vi "RobotOpen.vi"(8 "error in (no error)":errorcluster, 9 "RobotType":T1, 11 "Robot Communication port name":refnum<visa-resource-name>="ASRL2::INSTR") -> (0 "error out":errorcluster, 3 "Robot Communication port name out":refnum<visa-resource-name>)   [LabVIEW 2014]
doc: "Open UART serial port and initilize iRobot."
uses:
  RobotType.ctl
  <vilib>/myRIO/Instrument Drivers/Onboard IO/UART/typedef/VISA Configuration.ctl
  <vilib>/Instr/_visa.llb/VISA Flush IO Buffer Mask.ctl
  iRobot/Actuator/LED.ctl
  iRobot/Advanced/Command/Baud.ctl
  <vilib>/Instr/_visa.llb/VISA Configure Serial Port (Instr).vi
  <vilib>/myRIO/Instrument Drivers/Onboard IO/UART/UART.lvlib
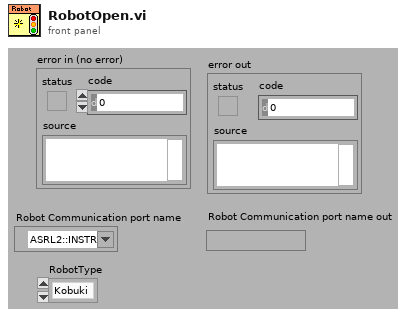
[diagram p1: front panel]
types:
  T1 = typedef "RobotType.ctl" = enum16{"Kobuki", "iRobot"}
  T2 = typedef "Baud.ctl" = enum8{"300", "600", "1200", "2400", "4800", "9600", "14400", "19200", "28800", "38400", "57600", "115200"}
  T3 = typedef "VISA Flush IO Buffer Mask.ctl" = u16
  T4 = typedef "UART.lvlib/VISA Configuration.ctl" = cluster{"baud rate (9600)":u32, "data bits (8)":u16, "parity (0:none)":enum16{"None", "Odd", "Even", "Mark", "Space"}, "stop bits (10: 1 bit)":u16, "flow control (0:none)":u16, "termination char\n(0xA = '\\n' = LF) ":u8, "Enable Termination\nChar (T)":bool, "timeout (10sec)":u32}
  T5 = typedef "LED.ctl" = u8
  T6 = typedef "iRobot UART Port Type.ctl" = refnum<visa-resource-name>
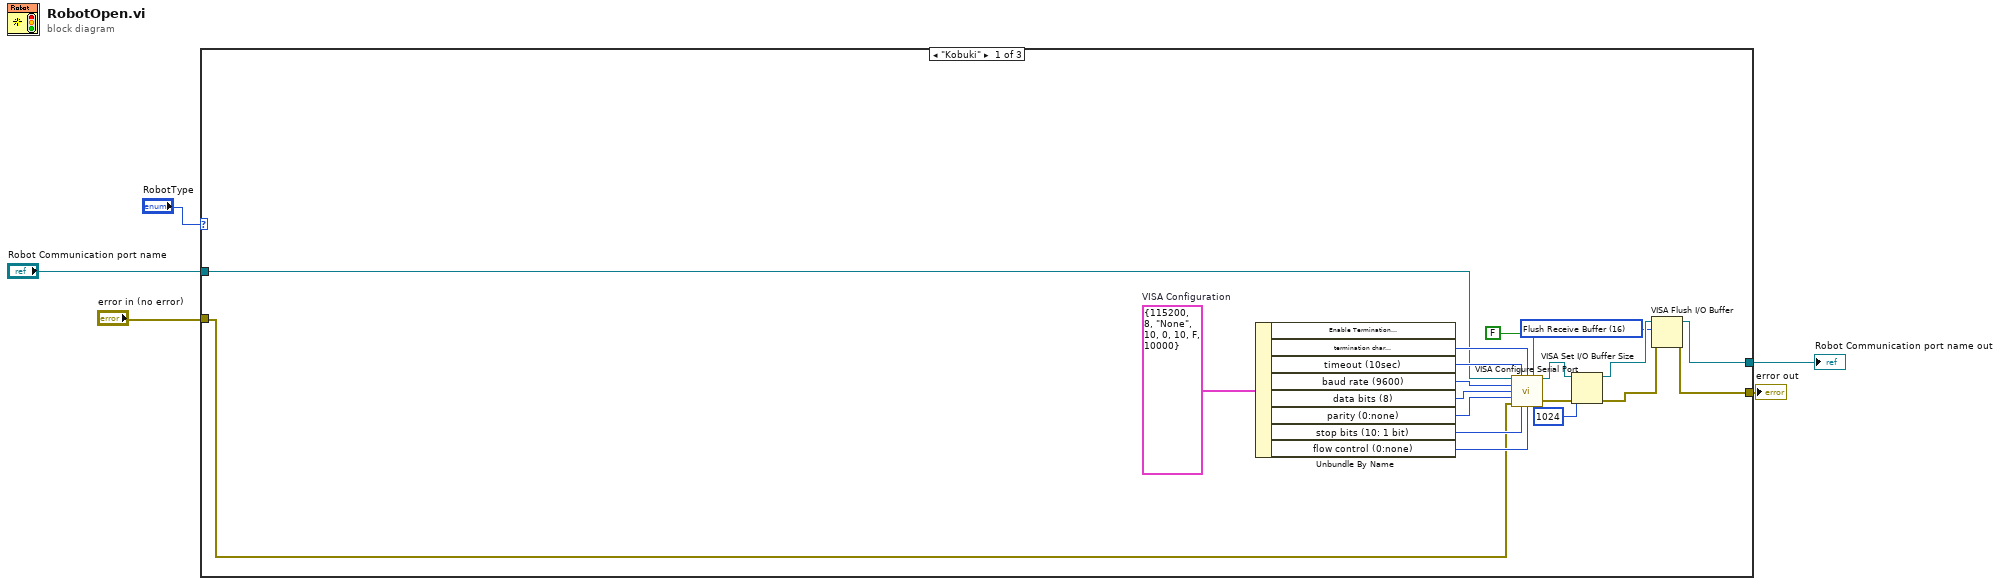
[diagram p0: block diagram]
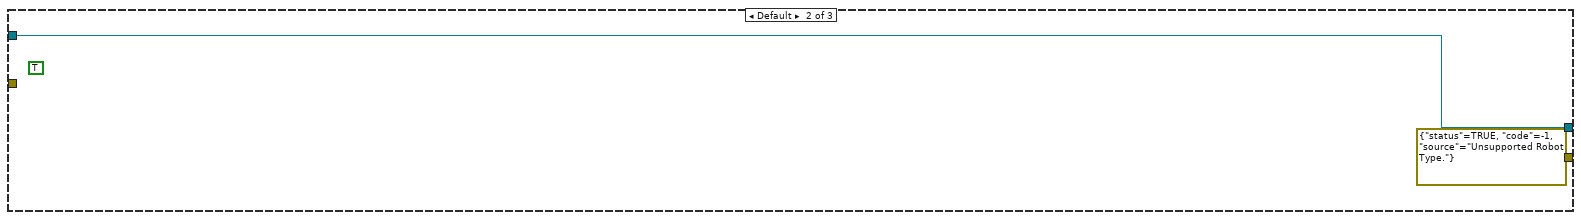
[diagram p2: hidden frame]
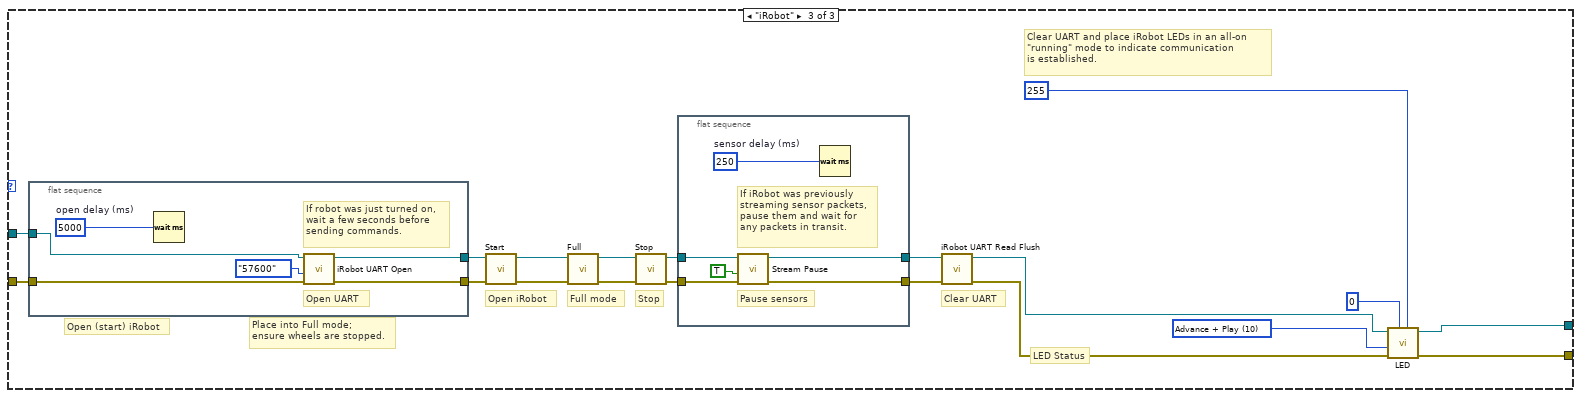
[diagram p3: hidden frame]
diagram:
  n1 = case shown="\"Kobuki\"" "RobotType" {
    tunnel: [w8 w26 w45] -> w1
    tunnel: [w6 errorcluster {"status"=TRUE, "code"=-1, "source"="Unsupported Robot Type."} ("error out") w44] -> w5
    tunnel: "error in (no error)" -> [w12 _ w43]
    tunnel: "Robot Communication port name" -> [w15 w26 w27]
    frame "Kobuki" {
      w9 = T3 16 items=["Flush Receive Buffer"=16, "Write Transmit Buffer to Device"=32, "Flush Receive Buffer (No I/O)"=64, "Flush Transmit Buffer"=128] ("Mask")
      w24 = T4 {"baud rate (9600)"=115200, "data bits (8)"=8, "parity (0:none)"=enum."None", "stop bits (10: 1 bit)"=10, "flow control (0:none)"=0, "termination char\n(0xA = '\\n' = LF) "=10, "Enable Termination\nChar (T)"=FALSE, "timeout (10sec)"=10000}  # VISA Configuration
      n2 = Unbundle By Name(w24) -> ("termination char\n(0xA = '\\n' = LF)"=w23:u8, "timeout (10sec)"=w22:u32, "baud rate (9600)"=w17:u32, "data bits (8)"=w18:u16, "parity (0:none)"=w19:enum16{"None", "Odd", "Even", "Mark", "Space"}, "stop bits (10: 1 bit)"=w20:u16, "flow control (0:none)"=w21:u16)  [unwired: 1 out]
      n3 = call-poly "VISA Configure Serial Port"("VISA resource name"=w15, "timeout (10sec)"=w22, "termination char\n(0xA = '\\n' = LF)"=w23, "Enable Termination\nChar (T)"=FALSE ("Enable Termination\nChar (T)"), "baud rate (9600)"=w17, "data bits (8)"=w18, "parity (0:none)"=w19, "error in (no error)"=w12, "stop bits (10: 1 bit)"=w20, "flow control (0:none)"=w21) -> ("VISA resource name out"=w14:refnum<visa-resource-name>, "error out"=w13:errorcluster)  [unwired: 4 in]
      n4 = VISA Set I/O Buffer Size(VISA resource name=w14, size (4096)=u32 1024, error in (no error)=w13) -> (VISA resource name out=w10:refnum<visa-resource-name>, error out=w7:errorcluster)  [unwired: 1 in]
      n5 = VISA Flush I/O Buffer(VISA resource name=w10, mask (16)=w9, error in (no error)=w7) -> (VISA resource name out=w8:refnum<visa-resource-name>, error out=w6:errorcluster)
    }
    frame Default {
      (unwired) TRUE ("status")
    }
    frame "iRobot" {
      w31 = T5 10 items=["None"=0, "Advance"=8, "Play"=2, "Advance + Play"=10] ("LEDs on")
      # "Clear UART and place iRobot LEDs in an all-on\n\"running\" mode to indicate communication\nis established."
      # "Clear UART"
      # "LED Status"
      # "Place into Full mode;\nensure wheels are stopped."
      # "Full mode"
      # "Stop"
      # "Open (start) iRobot"
      # "Open iRobot"
      n6 = flat-sequence {
        tunnel: [w57] -> w38
        tunnel: [w56] -> w36
        tunnel: w43 -> [w53]
        tunnel: w27 -> [w52]
        frame #0 {
          w55 = u32 5000  # open delay (ms)
          # "If robot was just turned on,\nwait a few seconds before\nsending commands."
          # "Open UART"
          n7 = Wait (ms)(milliseconds to wait=w55) -> ()  [unwired: 1 out]
          n8 = call "iRobot UART Open.vi"("error in (no error)"=w53, "Baud Rate (BPS)"=Baud."57600", "UART port in"=w52) -> ("error out"=w56:errorcluster, "UART port out"=w57:T6)  [unwired: 7 out]
        }
      }
      n9 = call "Start.vi"("error in"=w36, "UART port in"=w38) -> ("error out"=w35:errorcluster, "UART port out"=w37:T6)  [unwired: 8 out]
      n10 = call "Full.vi"("error in"=w35, "UART port in"=w37) -> ("error out"=w33:errorcluster, "UART port out"=w34:T6)  [unwired: 8 out]
      n11 = call "Stop.vi"("error in"=w33, "UART port in"=w34) -> ("error out"=w40:errorcluster, "UART port out"=w41:T6)  [unwired: 8 out]
      n12 = flat-sequence {
        tunnel: [w51] -> w42
        tunnel: w41 -> [w50]
        tunnel: w40 -> [w49]
        tunnel: [w48] -> w39
        frame #0 {
          w47 = u32 250  # sensor delay (ms)
          # "If iRobot was previously\nstreaming sensor packets,\npause them and wait for\nany packets in transit."
          # "Pause sensors"
          n13 = call "Stream Pause.vi"("error in"=w49, "Pause?"=TRUE ("Resume?"), "UART port in"=w50) -> ("error out"=w48:errorcluster, "UART port out"=w51:T6)  [unwired: 1 in, 6 out]
          n14 = Wait (ms)(milliseconds to wait=w47) -> ()  [unwired: 1 out]
        }
      }
      n15 = call "iRobot UART Read Flush.vi"("error in"=w39, "UART port in"=w42) -> ("error out"=w30:errorcluster, "UART port out"=w32:T6)  [unwired: 8 out]
      n16 = call "LED.vi"("Power LED Intensity (0-255)"=u8 255 ("Power LED Color (R-G)"), "Power LED Color (G[0]-R[255])"=u8 0, "error in"=w30, "LEDs on"=w31, "UART port in"=w32) -> ("error out"=w44:errorcluster, "UART port out"=w45:T6)  [unwired: 3 in, 2 out]
    }
  }
  "error out" <- w5
  "Robot Communication port name out" <- w1
